vi "2D Points Path to 2D Points Trajectory.vi"() -> ()   [LabVIEW 2015]
panel:
  out "Index":i32
  out "Robot Position":cluster{dbl[], dbl[]}[](graph)
  out "Total Time":dbl
  in  "Max Speed (dx/dt)":dbl=3.0
  in  "dt/1000,  milliseconds!!!":dbl=10.0
  out "Final Position":dbl
  out "acceleration [x/t^2]":dbl[](array[numeric])
  out "Position [x]":dbl[](array[numeric])
  out "velocity [x/t]":dbl[](array[numeric])
  out "XY Graph":cluster{dbl[], dbl[]}[](graph)
  in  "Max Jerk (dx/dt3)":dbl=1.0
  in  "Max Acceleration (dx/dt^2)":dbl=1.0
  in  "Points":T1(array[cluster])
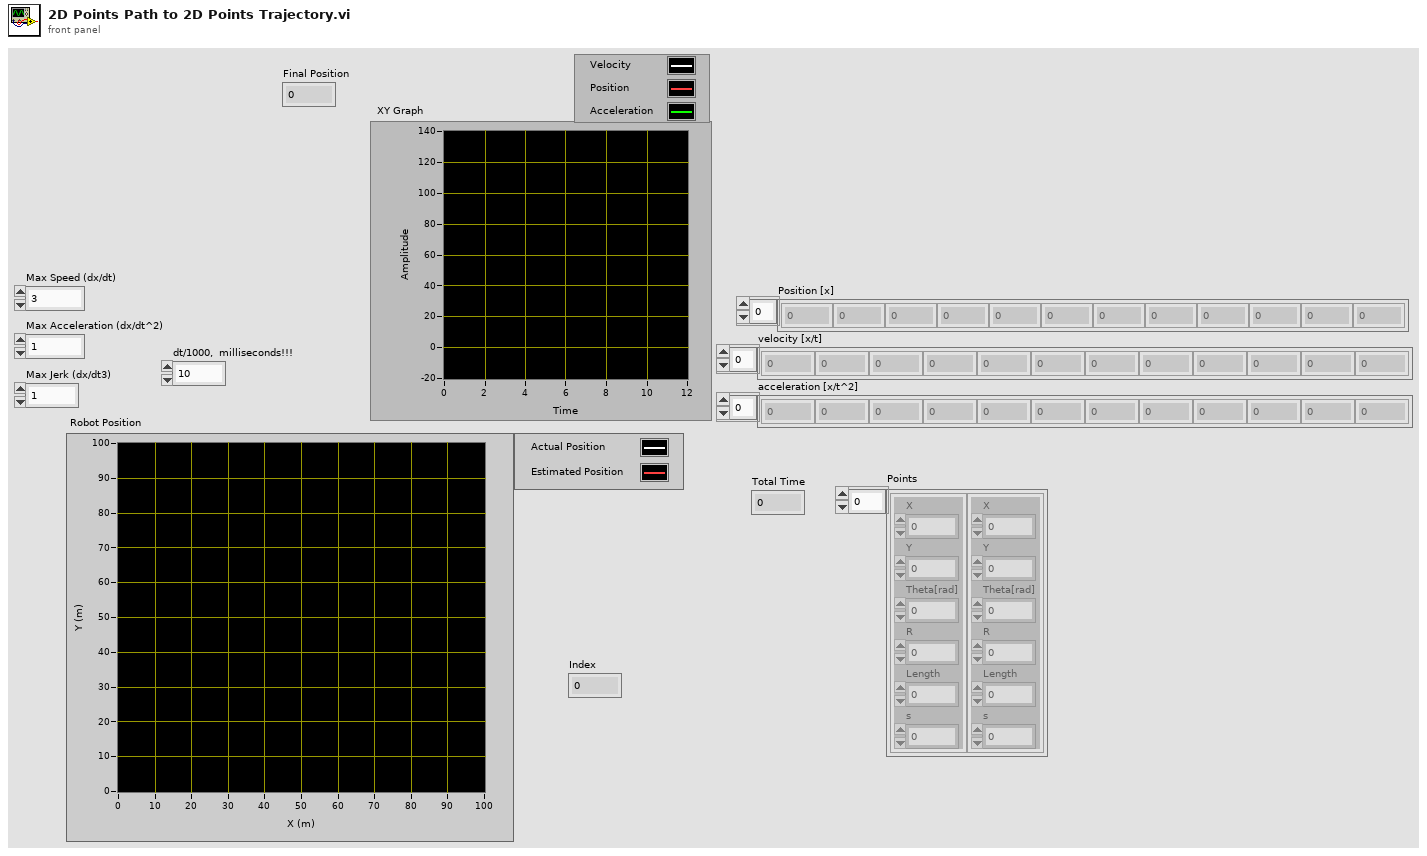
[diagram p1: front panel]
types:
  T1 = cluster{"X":dbl, "Y":dbl, "Theta[rad]":dbl, "R":dbl, "Length":dbl, "s":dbl}[]
  T2 = cluster{"X":dbl, "Y":dbl, "Theta[rad]":dbl, "R":dbl, "Length":dbl, "s":dbl}
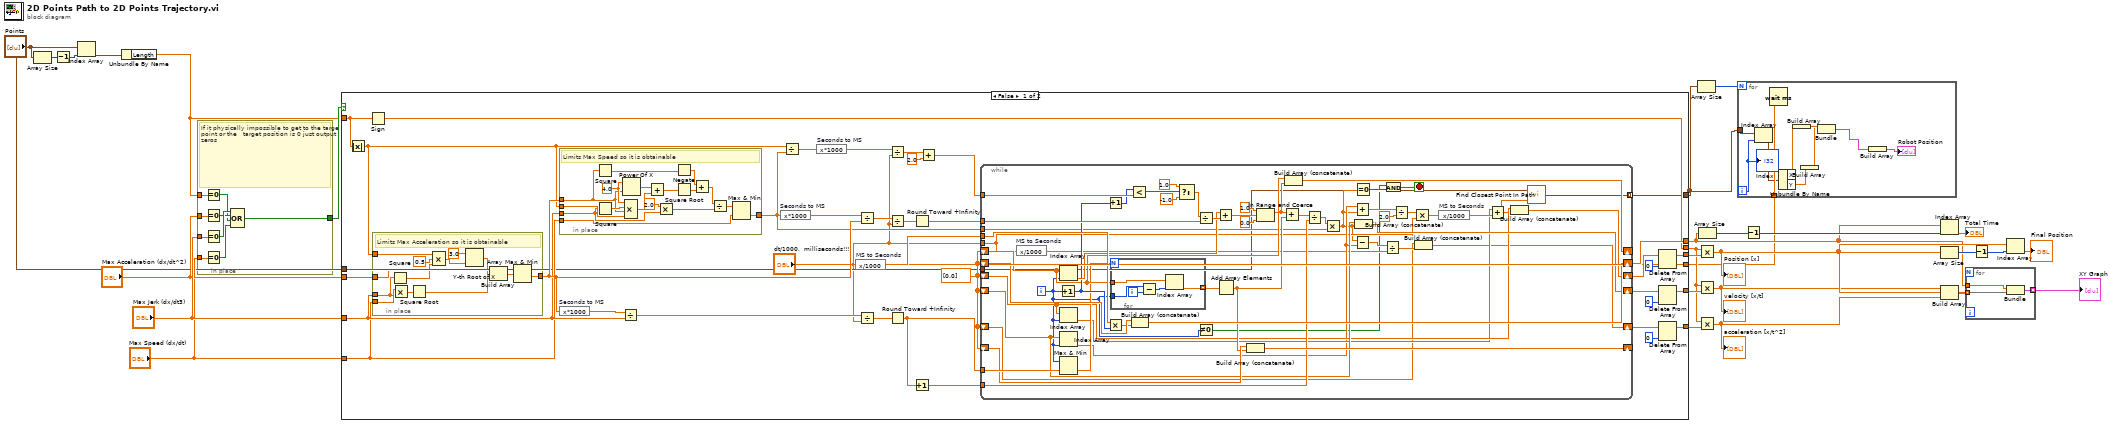
[diagram p0: block diagram]
diagram:
  n1 = Array Size(array="Points") -> (size(s)=w28:i32)
  n2 = Decrement(x=w28) -> (x-1=w27:i32)
  n3 = Index Array(array="Points", index=w27) -> (element=w26:T2)
  n4 = Unbundle By Name(w26) -> ("Length"=w5:dbl)
  n5 = in-place {
    in-place-border: "Max Jerk (dx/dt3)" -> [w37]
    in-place-border: "Max Acceleration (dx/dt^2)" -> [w36]
    in-place-border: w5 -> [w35]
    in-place-border: [w31] -> w15
    in-place-border: "Max Speed (dx/dt)" -> [w29]
    # "If it physically impossible to get to the target point or the   target position is 0 just output zeros"
    n6 = Equal To 0?(x=w35) -> (x = 0?=w32:bool)
    n7 = Equal To 0?(x=w36) -> (x = 0?=w33:bool)
    n8 = Equal To 0?(x=w37) -> (x = 0?=w34:bool)
    n9 = Equal To 0?(x=w29) -> (x = 0?=w30:bool)
    n10 = Compound Arithmetic op=OR(w34, w33, w32, w30) -> (w31:bool)
  }
  n11 = case shown="False" w15 {
    tunnel: [w59 _] -> w7
    tunnel: [w53 _] -> w20
    tunnel: [w49 _] -> w19
    tunnel: [w48 _] -> w18
    tunnel: "Max Jerk (dx/dt3)" -> [w47 _]
    tunnel: "Max Acceleration (dx/dt^2)" -> [w46 _]
    tunnel: w5 -> [w42 _]
    tunnel: "Max Speed (dx/dt)" -> [w44 _]
    tunnel: [w41 _] -> w10
    tunnel: "Points" -> [w40 _]
    tunnel: [w39 _] -> w1
    tunnel: ["dt/1000,  milliseconds!!!" _] -> w2
    frame False {
      w60 = dbl[] [0.0]
      n12 = Absolute Value(x=w42) -> (abs(x)=w43:dbl)
      n13 = Sign(1:w42) -> (0:w41:dbl)
      n14 = in-place {
        in-place-border: w47 -> [w78]
        in-place-border: w46 -> [w82]
        in-place-border: [w75] -> w58
        in-place-border: w43 -> [w87]
        in-place-border: w44 -> [w79]
        # "Limits Max Acceleration so it is obtainable"
        n15 = Square(x=w78) -> (x^2=w85:dbl)
        n16 = Multiply(x=w79, y=w78) -> (x*y=w80:dbl)
        n17 = Square Root(x=w80) -> (sqrt(x)=w77:dbl)
        n18 = Compound Arithmetic op=MULTIPLY(w87, 0.5 ("value"), w85) -> (w84:dbl)
        n19 = Y-th Root of X(1:w84, 2:3.0 ("y")) -> (0:w81:dbl)
        n20 = Build Array(w82, w81, w77) -> (w76:dbl[])
        n21 = Array Max & Min(array=w76) -> (min value=w75:dbl)  [unwired: 3 out]
      }
      n22 = in-place {
        in-place-border: w44 -> [w104]
        in-place-border: [w91] -> w57
        in-place-border: w58 -> [w97]
        in-place-border: w43 -> [w96]
        in-place-border: w47 -> [w93]
        w100 = 4.0 ("x")
        # "Limits Max Speed so it is obtainable"
        n23 = Square(x=w97) -> (x^2=w103:dbl)
        n24 = Square(x=w93) -> (x^2=w99:dbl)
        n25 = Power Of X(1:w97, 2:w100) -> (0:w101:dbl)
        n26 = Compound Arithmetic op=MULTIPLY(w100, w99, w97, w96) -> (w98:dbl)
        n27 = Add(x=w101, y=w98) -> (x+y=w95:dbl)
        n28 = Multiply(x=2.0, y=w93) -> (x*y=w88:dbl)
        n29 = Negate(x=w103) -> (-x=w102:dbl)
        n30 = Square Root(x=w95) -> (sqrt(x)=w92:dbl)
        n31 = Add(x=w102, y=w92) -> (x+y=w90:dbl)
        n32 = Divide(x=w90, y=w88) -> (x/y=w89:dbl)
        n33 = Max & Min(x=w89, y=w104) -> (min(x,y)=w91:dbl)  [unwired: 1 out]
      }
      n34 = expression code="x*1000" "Seconds to MS"(w58) -> (w73:dbl)
      n35 = Divide(x=w73, y=w47) -> (x/y=w45:dbl)
      n36 = expression code="x*1000" "Seconds to MS"(w57) -> (w72:dbl)
      n37 = Divide(x=w43, y=w57) -> (x/y=w71:dbl)
      n38 = expression code="x*1000" "Seconds to MS"(w71) -> (w70:dbl)
      n39 = expression code="x/1000" "MS to Seconds"("dt/1000,  milliseconds!!!") -> (w74:dbl)
      n40 = Divide(x=w72, y=w58) -> (x/y=w66:dbl)
      n41 = Divide(x=w45, y="dt/1000,  milliseconds!!!") -> (x/y=w63:dbl)
      n42 = Divide(x=w70, y="dt/1000,  milliseconds!!!") -> (x/y=w69:dbl)
      n43 = Divide(x=w66, y="dt/1000,  milliseconds!!!") -> (x/y=w65:dbl)
      n44 = Round Toward +Infinity(x=w63) -> (ceil(x): smallest int >= x=w62:dbl)
      n45 = Round Toward +Infinity(x=w65) -> (ceil(x): smallest int >= x=w64:dbl)
      n46 = Increment(x=w62) -> (x+1=w61:dbl)
      n47 = Add(x=w69, y=2.0) -> (x+y=w67:dbl)
      n48 = while {
        shift-right: [w158] -> w59
        shift-left: w60 -> [w159]
        tunnel: w74 -> [w157]
        tunnel: w67 -> [w155]
        shift-right: [w145] -> _
        shift-left: w60 -> [w144]
        tunnel: w64 -> [w150]
        tunnel: w62 -> [w142]
        shift-right: [w139] -> _
        shift-left: w60 -> [w140]
        tunnel: w61 -> [w136]
        tunnel: w57 -> [w134]
        shift-right: [w133] -> w52
        shift-left: w60 -> [w131]
        shift-right: [w132] -> w50
        shift-left: w60 -> [w125]
        tunnel: "dt/1000,  milliseconds!!!" -> [w120]
        shift-right: [w118] -> w54
        shift-left: w60 -> [w117]
        tunnel: w40 -> [w106]
        tunnel: [w105] -> w39 mode=indexing
        i -> [w116]
        stop <- w112 stop-if-true
        n49 = expression code="x/1000" "MS to Seconds"(w120) -> (w121:dbl)
        n50 = Index Array(array=w144, index=w116) -> (element=w148:dbl)
        n51 = Increment(x=w116) -> (x+1=w146:i32)
        n52 = Index Array(array=w125, index=w116) -> (element=w124:dbl)
        n53 = Index Array(array=w131, index=w116) -> (element=w123:dbl)
        n54 = Max & Min(x=w116, y=w142) -> (min(x,y)=w141:dbl)  [unwired: 1 out]
        n55 = Increment(x=w146) -> (x+1=w147:i32)
        n56 = Multiply(x=w157, y=w146) -> (x*y=w156:dbl)
        n57 = for {
          N: w141 -> [_]
          tunnel: w116 -> [w163]
          tunnel: w144 -> [w161]
          tunnel: [w160] -> w143 mode=indexing
          i -> [w164]
          n58 = Subtract(x=w163, y=w164) -> (x-y=w162:i32)
          n59 = Index Array(array=w161, index=w162) -> (element=w160:dbl)
        }
        n60 = Less?(x=w147, y=w155) -> (x < y?=w154:bool)
        n61 = Build Array (concatenate)(w159, w156) -> (w158:dbl[])
        n62 = Select(t=1.0, s=w154, f=-1.0) -> (s? t:f=w151:dbl)
        n63 = Divide(x=w151, y=w150) -> (x/y=w149:dbl)
        n64 = Not Equal To 0?(x=w116) -> (x != 0?=w113:bool)
        n65 = Add(x=w148, y=w149) -> (x+y=w109:dbl)
        n66 = Add Array Elements(numeric array=w143) -> (sum=w138:dbl)
        n67 = Build Array (concatenate)(w140, w138) -> (w139:dbl[])
        n68 = In Range and Coerce(upper limit=1.0, x=w109, lower limit=0.0) -> (coerced(x)=w108:dbl)  [unwired: 1 out]
        n69 = Add(x=w108, y=w138) -> (x+y=w137:dbl)
        n70 = Build Array (concatenate)(w144, w108) -> (w145:dbl[])
        n71 = Divide(x=w137, y=w136) -> (x/y=w135:dbl)
        n72 = Multiply(x=w135, y=w134) -> (x*y=w115:dbl)
        n73 = Add(x=w123, y=w115) -> (x+y=w130:dbl)
        n74 = Subtract(x=w115, y=w123) -> (x-y=w122:dbl)
        n75 = Equal To 0?(x=w115) -> (x = 0?=w114:bool)
        n76 = Build Array (concatenate)(w131, w115) -> (w133:dbl[])
        n77 = Divide(x=w122, y=w121) -> (x/y=w119:dbl)
        n78 = And(x=w113, y=w114) -> (x .and. y?=w112:bool)
        n79 = Divide(x=w130, y=2.0) -> (x/y=w128:dbl)
        n80 = Multiply(x=w128, y=w120) -> (x*y=w127:dbl)
        n81 = Build Array (concatenate)(w117, w119) -> (w118:dbl[])
        n82 = expression code="x/1000" "MS to Seconds"(w127) -> (w126:dbl)
        n83 = Add(x=w124, y=w126) -> (x+y=w107:dbl)
        n84 = Build Array (concatenate)(w125, w107) -> (w132:dbl[])
        n85 = call "Find Closest Point In Path.vi"("Length"=w107, "Points"=w106) -> ("Point"=w105:T2)
      }
      n86 = Delete From Array(array=w50, index=0) -> (array with subset deleted=w49:dbl[])  [unwired: 1 in, 1 out]
      n87 = Delete From Array(array=w52, index=0) -> (array with subset deleted=w48:dbl[])  [unwired: 1 in, 1 out]
      n88 = Delete From Array(array=w54, index=0) -> (array with subset deleted=w53:dbl[])  [unwired: 1 in, 1 out]
    }
    frame True {
    }
  }
  n89 = Array Size(array=w1) -> (size(s)=w3:i32)
  n90 = Multiply(x=w10, y=w19) -> (x*y=w13:dbl[])
  "Position [x]" <- w13
  n91 = Multiply(x=w10, y=w18) -> (x*y=w12:dbl[])
  "velocity [x/t]" <- w12
  n92 = Multiply(x=w10, y=w20) -> (x*y=w11:dbl[])
  "acceleration [x/t^2]" <- w11
  n93 = Array Size(array=w7) -> (size(s)=w9:i32)
  n94 = for {
    N: w3 -> [_]
    tunnel: w2 -> [w174]
    tunnel: w1 -> [w173]
    i -> [w172]
    n95 = Index Array(array=w173, index=w172) -> (element=w171:T2)
    n96 = Wait (ms)(milliseconds to wait=w174) -> ()  [unwired: 1 out]
    n97 = Unbundle By Name(w171) -> ("X"=w170:dbl, "Y"=w169:dbl)
    n98 = Build Array(w170) -> (w166:dbl[])
    n99 = Build Array(w169) -> (w165:dbl[])
    n100 = Bundle(w165, w166) -> (w167:cluster{dbl[], dbl[]})  [unwired: 1 in]
    n101 = Build Array(w167) -> (→"Robot Position":cluster{dbl[], dbl[]}[])
    "Index" <- w172
  }
  n102 = Decrement(x=w9) -> (x-1=w8:i32)
  n103 = Index Array(array=w7, index=w8) -> (element=→"Total Time":dbl)
  n104 = Array Size(array=w13) -> (size(s)=w23:i32)
  n105 = Build Array(w12, w13, w11) -> (w25:dbl[][])
  n106 = for {
    tunnel: w25 -> [w177] mode=indexing
    tunnel: w7 -> [w176]
    tunnel: [w175] -> w24 mode=indexing
    n107 = Bundle(w176, w177) -> (w175:cluster{dbl[], dbl[]})  [unwired: 1 in]
  }
  "XY Graph" <- w24
  n108 = Decrement(x=w23) -> (x-1=w22:i32)
  n109 = Index Array(array=w13, index=w22) -> (element=→"Final Position":dbl)
